vi "Framework Host Sobot.vi"() -> ()   [LabVIEW 2017]
uses:
  TypeDefinitions/TCP Cluster.ctl
  TypeDefinitions/TCP Commands.ctl
  AT901 API/TypeDefinitions/ES_ReflectorType.ctl
  AT901 API/Structures/Struct SystemUnits.ctl
  AT901 API/TypeDefinitions/ES_LengthUnit.ctl
  AT901 API/TypeDefinitions/ES_AngleUnit.ctl
  AT901 API/TypeDefinitions/ES_TemperatureUnit.ctl
  AT901 API/TypeDefinitions/ES_PressureUnit.ctl
  AT901 API/TypeDefinitions/ES_HumidityUnit.ctl
  AT901 API/Structures/Struct EnvironmentData.ctl
  AT901 API/TypeDefinitions/ES_MeasMode.ctl
  AT901 API/TypeDefinitions/ES_CoordinateSystemType.ctl
  AT901 API/Structures/Struct ContinuousTimeModeData.ctl
  AT901 API/TypeDefinitions/ES_RegionType.ctl
  TypeDefinitions/Events.ctl
  <vilib>/Utility/inputDevices.llb/closeJoystick.vi
panel:
  in  "ContinuousTimeModeData":T1={"TimeSeparation"=100, "NumberOfPoints"=0, "UseRegion"=FALSE, "ES_RegionType"=enum."ES_RT_Sphere"}
  in  "Tab Control":enum32{"Allgemein", "Lasertracker"}(tab)
  in  "Button 1":bool
  in  "Button 2":bool
  in  "Manual Drive":bool
  in  "Device Index":i32
  in  "Stop":bool
  out "Send":T3={"Datatype"=enum."Message", "String"="Send to sobot"}
  out "Receive":T3={"Datatype"=enum."Message", "String"="Send to sobot"}
  in  "LT SingleMeasurement":bool
  in  "LT Initialize":bool
  in  "LT GoBirdBath":bool
  in  "LT GetEnvParams":bool
  out "Environmental Data":T5
  in  "LT_SystemUnits":T6
  in  "ES ReflectorType":T12=enum."CCR - 1,5 in"
  in  "LT PowerLock":bool
  out "LT PowerLock Status":bool
  in  "ES_MeasMode":T13
  in  "ES_CoordinateSystemType":T14
  out "Meas Result":dbl[](array[numeric])
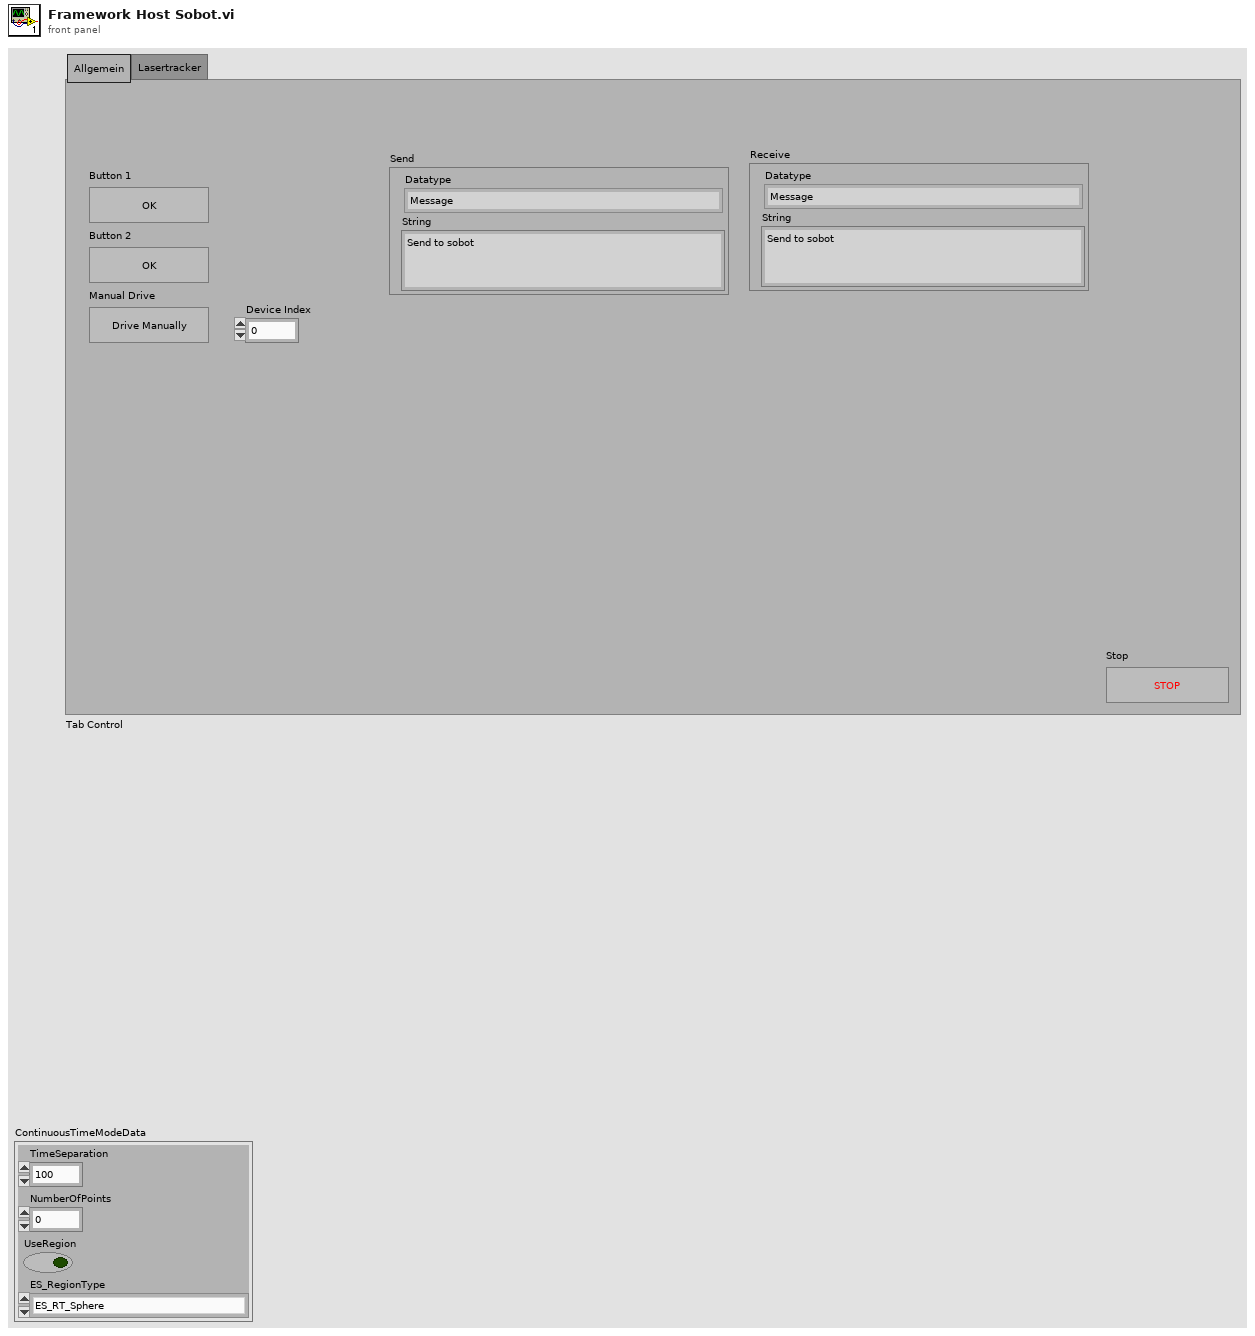
[diagram p1: front panel]
types:
  T1 = typedef "Struct ContinuousTimeModeData.ctl" = cluster{"TimeSeparation":u32, "NumberOfPoints":u32, "UseRegion":bool, "ES_RegionType":T2}
  T2 = typedef "ES_RegionType.ctl" = enum32{"ES_RT_Sphere", "ES_RT_Box"}
  T3 = typedef "TCP Cluster.ctl" = cluster{"Datatype":T4, "String":string}
  T4 = typedef "TCP Commands.ctl" = enum16{"Timeout", "Log", "Message", "ManualDrive", "Stop", "Command"}
  T5 = typedef "Struct EnvironmentData.ctl" = cluster{"Temperature":dbl, "Pressure":dbl, "Humidity":dbl}
  T6 = typedef "Struct SystemUnits.ctl" = cluster{"ES_LengthUnit":T7, "ES_AngleUnit":T8, "ES_TemperatureUnit":T9, "ES_PressureUnit":T10, "ES_HumidityUnit":T11}
  T7 = typedef "ES_LengthUnit.ctl" = enum32{"ES_LU__Meter", "ES_LU_Millimeter", "ES_LU_Micron", "ES_LU_Foot", "ES_LU_Yard", "ES_LU_Inch"}
  T8 = typedef "ES_AngleUnit.ctl" = enum32{"ES_AU_Radian", "ES_AU_Degree", "ES_AU_Gon"}
  T9 = typedef "ES_TemperatureUnit.ctl" = enum32{"ES_TU_Celsius", "ES_TU_Fahrenheit"}
  T10 = typedef "ES_PressureUnit.ctl" = enum32{"ES_PU_Mbar", "ES_PU_HPascal", "ES_PU_KPascal", "ES_PU_MmHg", "ES_PU_Psi", "ES_PU_InH2O", "ES_PU_InHg"}
  T11 = typedef "ES_HumidityUnit.ctl" = enum32{"ES_HU_RH"}
  T12 = typedef "ES_ReflectorType.ctl" = enum32{"none1", "none2", "CCR - 1,5 in", "none4", "none5", "TBR - 0,5 in", "none7", "CCR - 75mm", "none8", "RRR - 1,5 in"}
  T13 = typedef "ES_MeasMode.ctl" = enum32{"ES_MM_Stationary", "ES_MM_ContinuousTime", "ES_MM_ContinuousDistance", "ES_MM_Grid", "ES_MM_SphrereCenter", "ES_MM_CircleCenter", "ES_MM_6DStationary", "ES_MM_6DContinuousTime", "ES_MM_6DContinuousDistance", "ES_MM_6DGrid", "ES_MM_6DSphrereCenter", "ES_MM6DCircleCenter"}
  T14 = typedef "ES_CoordinateSystemType.ctl" = enum32{"ES_CS_RHR", "ES_CS_LHRX", "ES_CS_LHRY", "ES_CS_LHRZ", "ES_CS_CCW", "ES_CS_CCC", "ES_CS_SCW", "ES_CS_SCC"}
  T15 = typedef "Events.ctl" = enum16{"Timeout", "Stop", "Button 1", "Button 2", "StartManualDrive", "ManualDrive", "StopManualDrive", "LT_Initialize", "LT GoBirdBath", "LT_SetReflectorType", "LT_SystemUnits", "LT GetEnvParams", "LT PowerLock", "LT SetMeasMode", "LT SetCoordinateSystemType", "LT SingleMeasurement", "LT SetContinuousTimeModeData"}
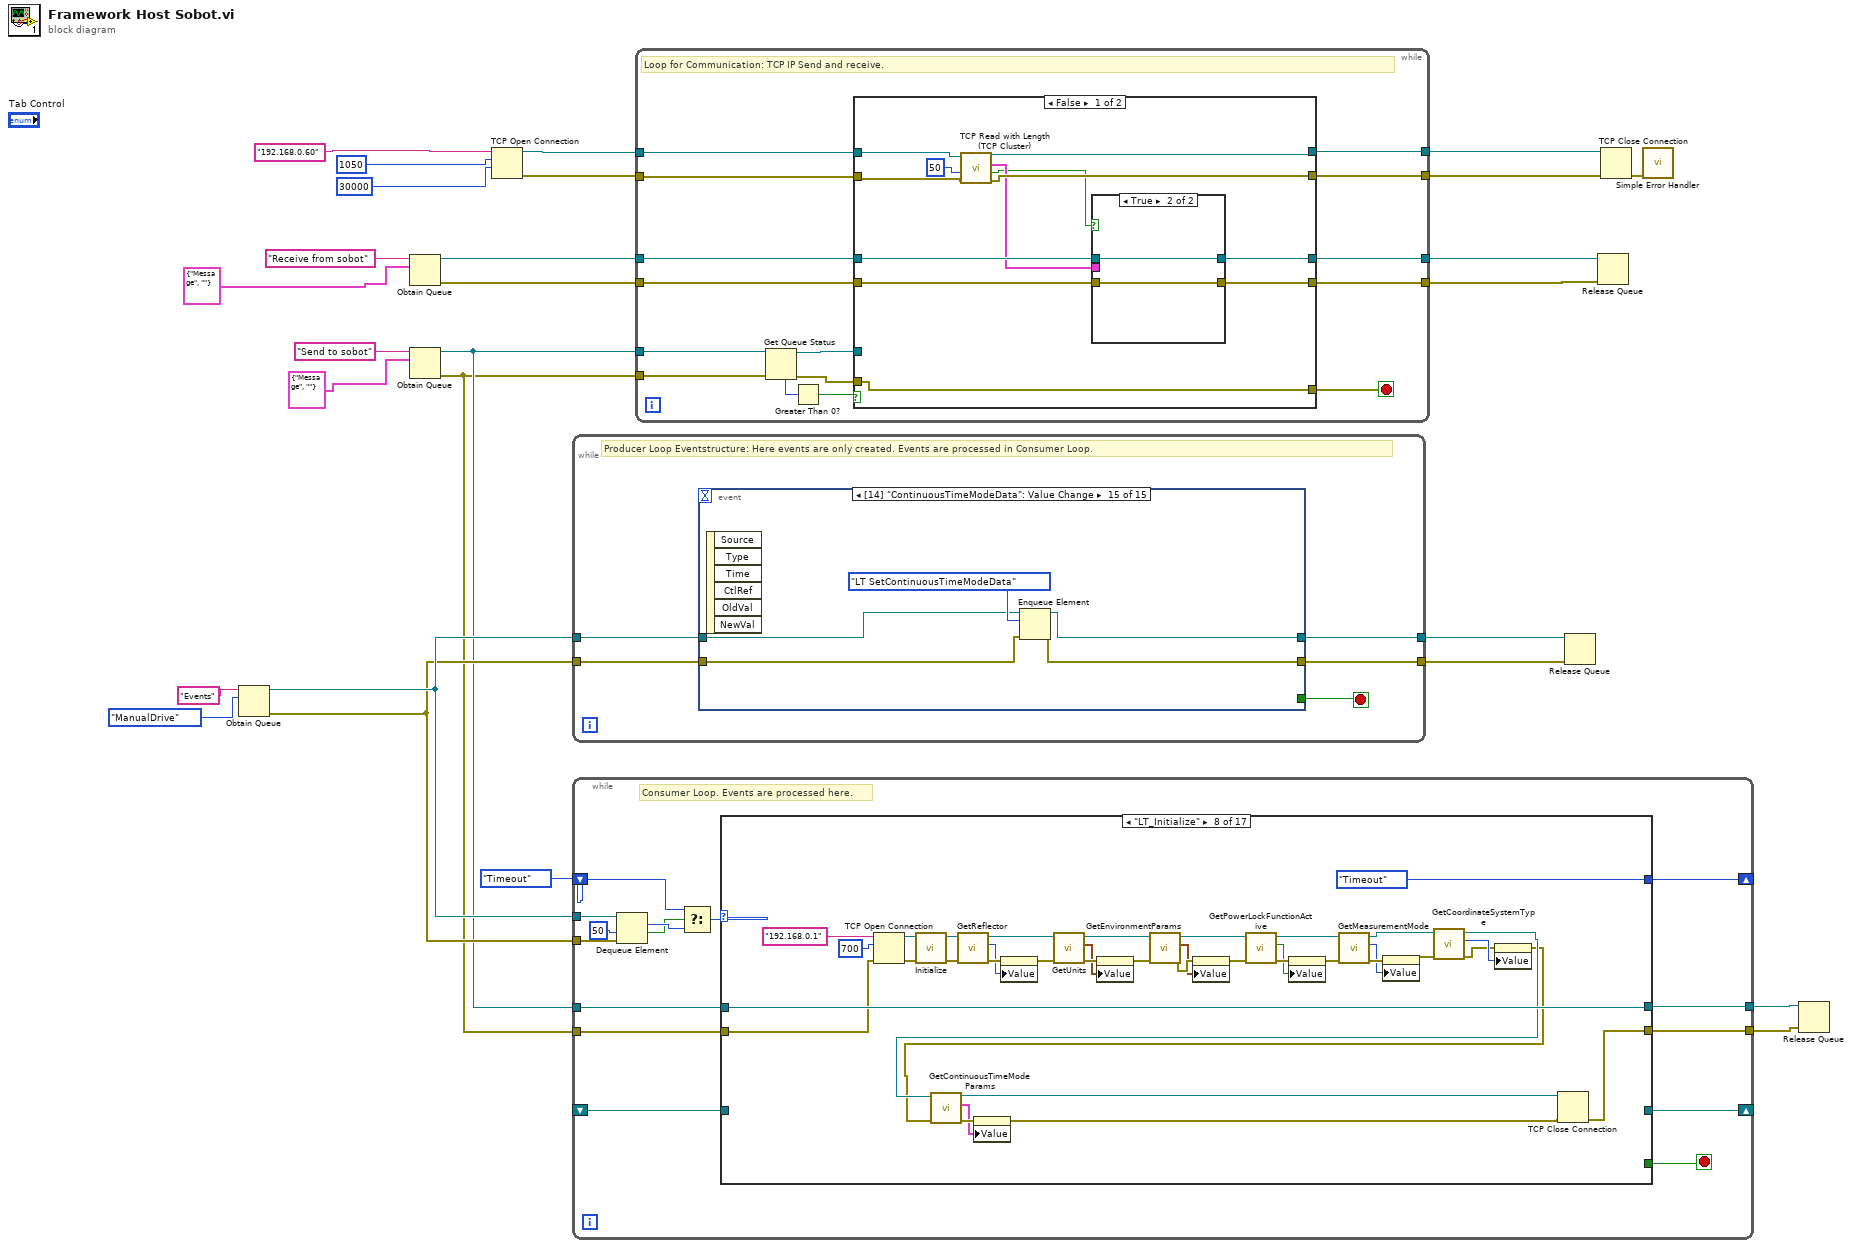
[diagram p0: block diagram]
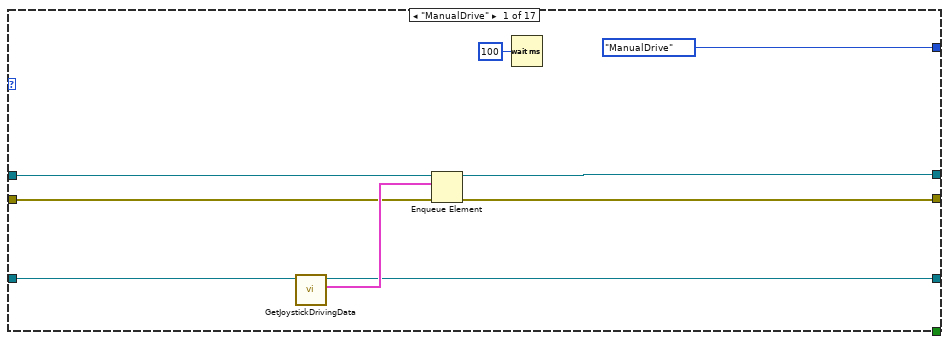
[diagram p2: hidden frame]
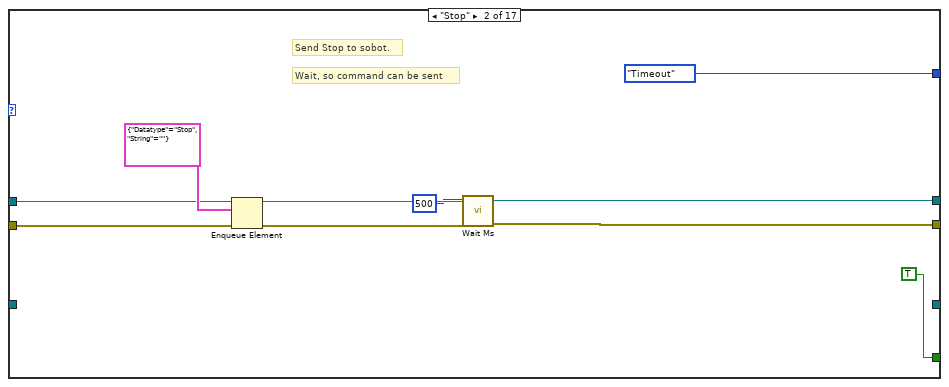
[diagram p3: hidden frame]
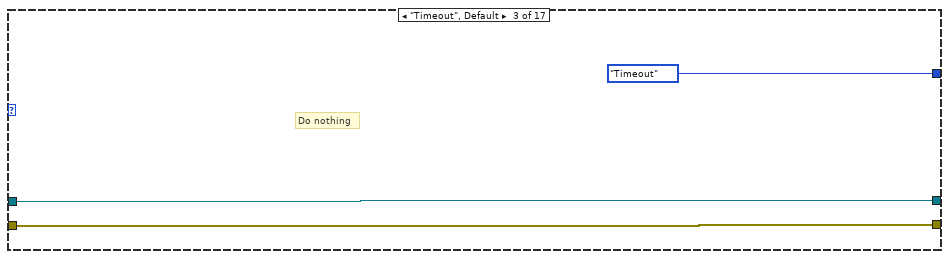
[diagram p4: hidden frame]
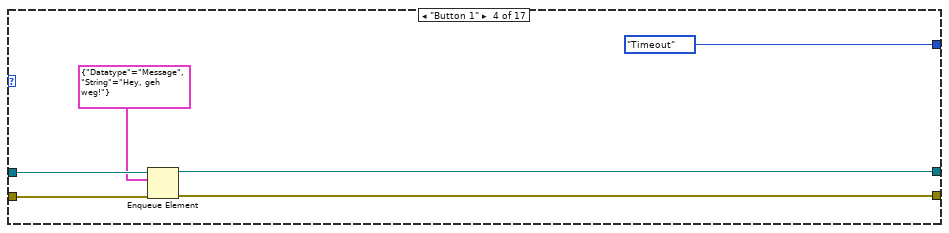
[diagram p5: hidden frame]
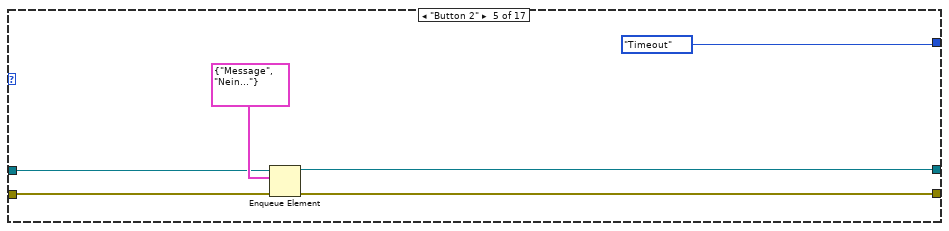
[diagram p6: hidden frame]
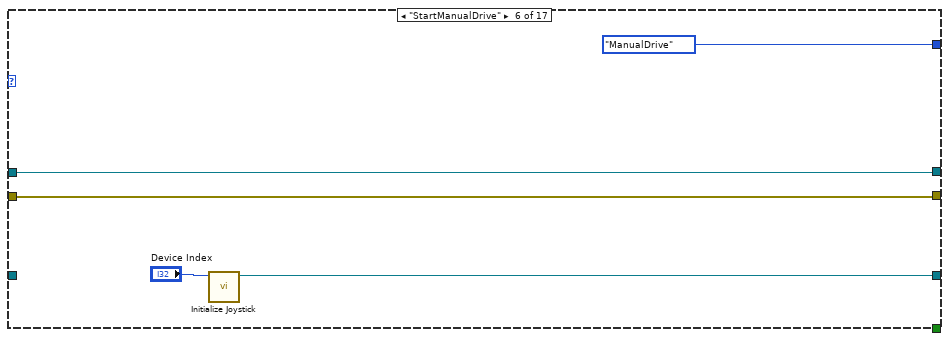
[diagram p7: hidden frame]
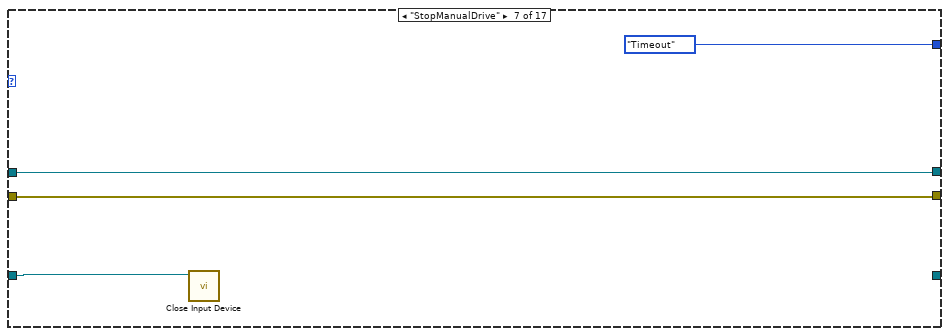
[diagram p8: hidden frame]
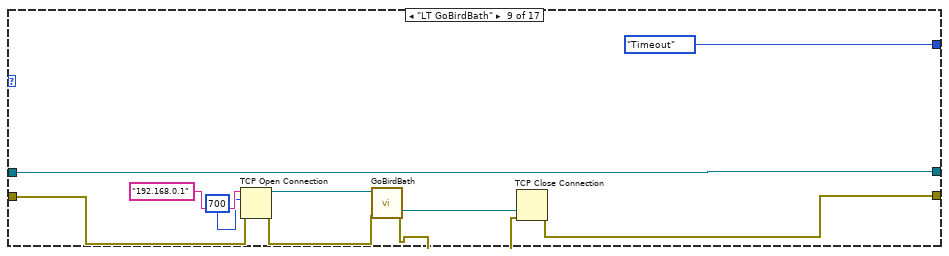
[diagram p9: hidden frame]
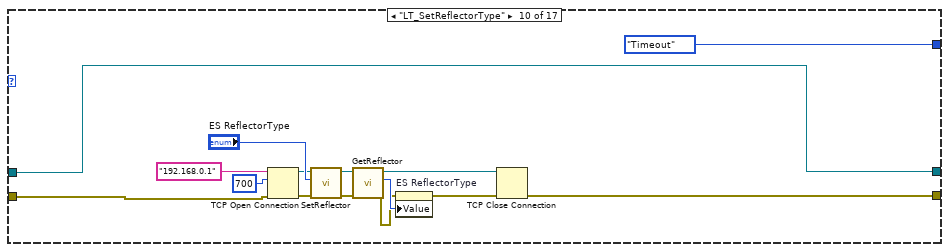
[diagram p10: hidden frame]
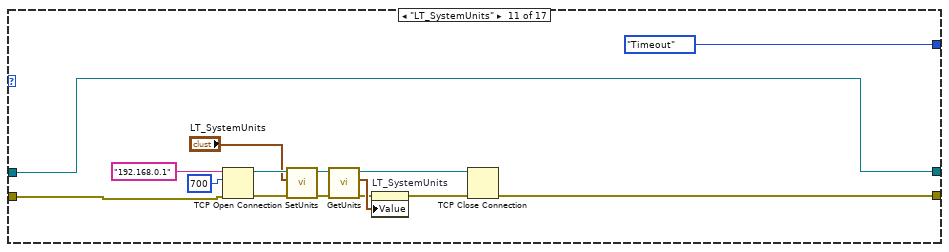
[diagram p11: hidden frame]
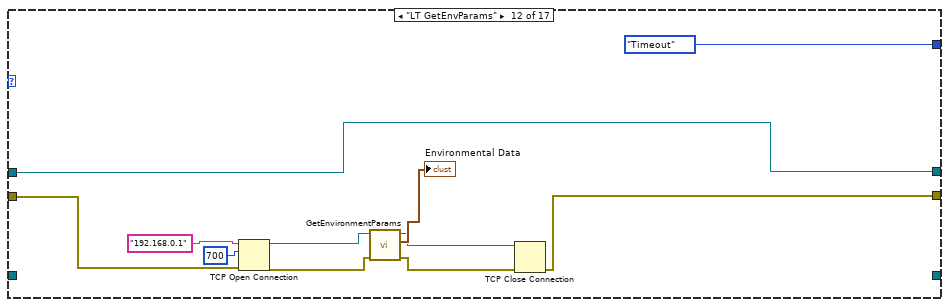
[diagram p12: hidden frame]
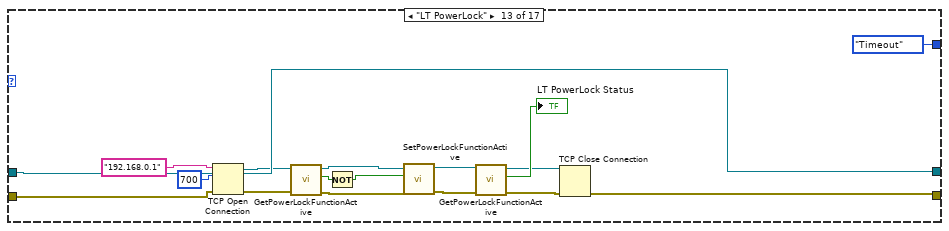
[diagram p13: hidden frame]
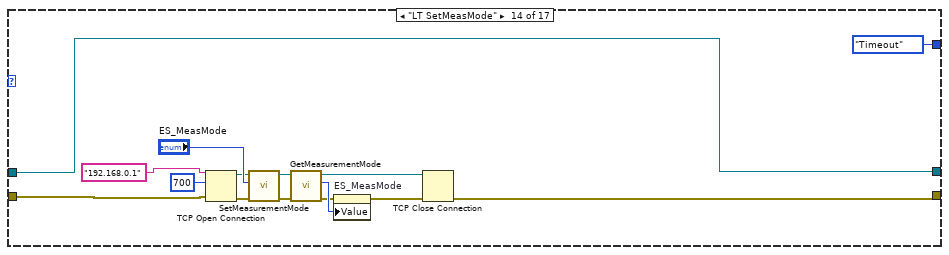
[diagram p14: hidden frame]
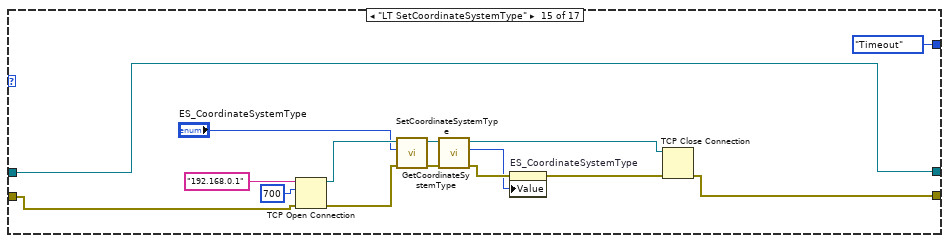
[diagram p15: hidden frame]
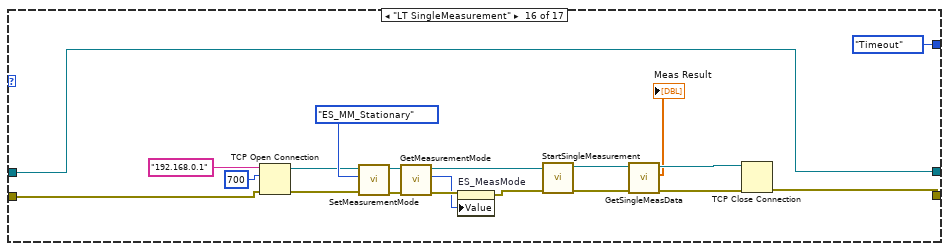
[diagram p16: hidden frame]
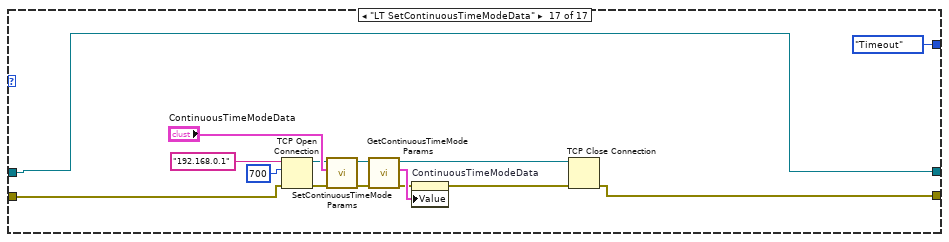
[diagram p17: hidden frame]
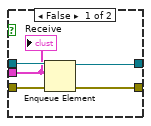
[diagram p18: hidden frame]
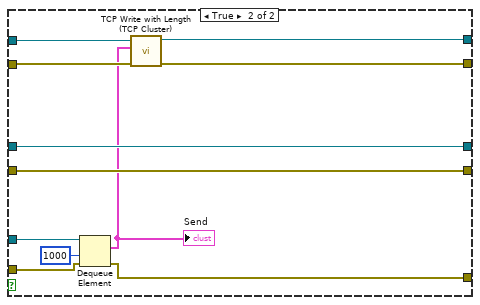
[diagram p19: hidden frame]
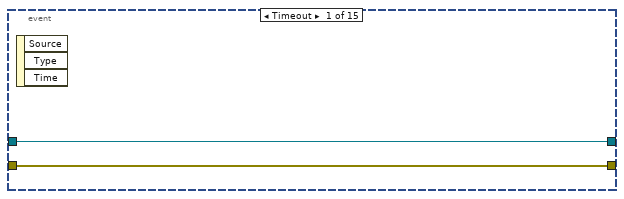
[diagram p20: hidden frame]
diagram:
  n1 = Obtain Queue(name (unnamed)="Events", element data type=Events."ManualDrive" ("Events")) -> (queue out=w7:refnum<queue>, error out=w6:errorcluster)  [unwired: 3 in, 1 out]
  n2 = Obtain Queue(name (unnamed)="Receive from sobot", element data type=T3 {"Datatype"=enum."Message", "String"=""}) -> (queue out=w22:refnum<queue>, error out=w21:errorcluster)  [unwired: 3 in, 1 out]
  n3 = Obtain Queue(name (unnamed)="Send to sobot", element data type=T3 {"Datatype"=enum."Message", "String"=""}) -> (queue out=w4:refnum<queue>, error out=w1:errorcluster)  [unwired: 3 in, 1 out]
  n4 = TCP Open Connection(address="192.168.0.60", remote port or service name=u16 1050, timeout ms (60000)=30000) -> (connection ID=w16:refnum<k5>, error out=w15:errorcluster)  [unwired: 2 in]
  n5 = while {
    tunnel: w7 -> [w31]
    tunnel: w6 -> [w30]
    tunnel: [w29] -> w9
    tunnel: [w28] -> w8
    stop <- w32 stop-if-true
    # "Producer Loop Eventstructure: Here events are only created. Events are processed in Consumer Loop."
    n6 = event shown="[14] \"ContinuousTimeModeData\": Value Change" {
      selector: _ -> [_ _ _ _ _ _ _ _ _ _ _ _ _ _ _]
      dyn-events: _ -> [_ _ _ _ _ _ _ _ _ _ _ _ _ _ _]
      timeout: _ -> [_ _ _ _ _ _ _ _ _ _ _ _ _ _ _]
      tunnel: [_ TRUE _ _ _ _ _ _ _ _ _ _ _ _ _] -> w32
      tunnel: w31 -> [w34 w43 w52 w55 w62 w67 w72 w77 w82 w87 w92 w97 w102 w106 w111]
      tunnel: w30 -> [w33 w41 w51 w56 w61 w66 w71 w76 w79 w86 w91 w96 w101 w105 w108]
      tunnel: [w34 w35 w50 w54 w60 w65 w70 w75 w81 w85 w89 w94 w99 w103 w110] -> w29
      tunnel: [w33 w36 w49 w53 w59 w64 w69 w74 w80 w84 w90 w93 w98 w104 w109] -> w28
      event Timeout {
        n7 = event-data() -> ()  [unwired: 1 in, 3 out]
      }
      event "Stop": Value Change {
        n8 = event-data() -> ()  [unwired: 1 in, 1 out]
        n9 = Enqueue Element(queue=w43, element=Events."Stop" ("Events"), error in (no error)=w41) -> (queue out=w35:refnum<queue>, error out=w39:errorcluster)  [unwired: 1 in, 1 out]
        n10 = call "Wait Ms.vi"("error in (no error)"=w39, "milliseconds to wait"=u32 500) -> ("error out"=w37:errorcluster)  [unwired: 9 in]
        n11 = property on="Stop" class="Bool (strict)"(error in=w37, "Value"=FALSE ("stop")) -> (error out=w36:errorcluster)  [unwired: 1 in, 1 out]
      }
      event "Manual Drive": Value Change {
        n12 = event-data() -> ("OldVal"=w48:bool)  [unwired: 1 in]
        n13 = Select(t=Events."StopManualDrive" ("Events"), s=w48, f=Events."StartManualDrive" ("Events")) -> (s? t:f=w46:T15)
        n14 = Enqueue Element(queue=w52, element=w46, error in (no error)=w51) -> (queue out=w50:refnum<queue>, error out=w49:errorcluster)  [unwired: 1 in, 1 out]
      }
      event "Button 1": Value Change {
        # "Send Example Message"
        n15 = event-data() -> ()  [unwired: 1 in, 1 out]
        n16 = Enqueue Element(queue=w55, element=Events."Button 1" ("Events"), error in (no error)=w56) -> (queue out=w54:refnum<queue>, error out=w53:errorcluster)  [unwired: 1 in, 1 out]
      }
      event "Button 2": Value Change {
        n17 = event-data() -> ()  [unwired: 1 in, 1 out]
        n18 = Enqueue Element(queue=w62, element=Events."Button 2" ("Events"), error in (no error)=w61) -> (queue out=w60:refnum<queue>, error out=w59:errorcluster)  [unwired: 1 in, 1 out]
      }
      event "LT Initialize": Value Change {
        n19 = event-data() -> ()  [unwired: 1 in, 1 out]
        n20 = Enqueue Element(queue=w67, element=Events."LT_Initialize", error in (no error)=w66) -> (queue out=w65:refnum<queue>, error out=w64:errorcluster)  [unwired: 1 in, 1 out]
      }
      event "LT GoBirdBath": Value Change {
        n21 = event-data() -> ()  [unwired: 1 in, 2 out]
        n22 = Enqueue Element(queue=w72, element=Events."LT GoBirdBath" ("Events"), error in (no error)=w71) -> (queue out=w70:refnum<queue>, error out=w69:errorcluster)  [unwired: 1 in, 1 out]
      }
      event Value Change {
        n23 = event-data() -> ()  [unwired: 1 in, 6 out]
        n24 = Enqueue Element(queue=w77, element=Events."LT_SetReflectorType" ("Events"), error in (no error)=w76) -> (queue out=w75:refnum<queue>, error out=w74:errorcluster)  [unwired: 1 in, 1 out]
      }
      event Value Change {
        n25 = event-data() -> ()  [unwired: 1 in, 6 out]
        n26 = Enqueue Element(queue=w82, element=Events."LT_SystemUnits" ("Events"), error in (no error)=w79) -> (queue out=w81:refnum<queue>, error out=w80:errorcluster)  [unwired: 1 in, 1 out]
      }
      event "LT GetEnvParams": Value Change {
        n27 = event-data() -> ()  [unwired: 1 in, 1 out]
        n28 = Enqueue Element(queue=w87, element=Events."LT GetEnvParams" ("Events"), error in (no error)=w86) -> (queue out=w85:refnum<queue>, error out=w84:errorcluster)  [unwired: 1 in, 1 out]
      }
      event "LT PowerLock": Value Change {
        n29 = event-data() -> ()  [unwired: 1 in, 2 out]
        n30 = Enqueue Element(queue=w92, element=Events."LT PowerLock" ("Events"), error in (no error)=w91) -> (queue out=w89:refnum<queue>, error out=w90:errorcluster)  [unwired: 1 in, 1 out]
      }
      event "LT SingleMeasurement": Value Change {
        n31 = event-data() -> ()  [unwired: 1 in, 1 out]
        n32 = Enqueue Element(queue=w97, element=Events."LT SingleMeasurement", error in (no error)=w96) -> (queue out=w94:refnum<queue>, error out=w93:errorcluster)  [unwired: 1 in, 1 out]
      }
      event Value Change {
        n33 = event-data() -> ()  [unwired: 1 in, 1 out]
        n34 = Enqueue Element(queue=w102, element=Events."LT SetMeasMode", error in (no error)=w101) -> (queue out=w99:refnum<queue>, error out=w98:errorcluster)  [unwired: 1 in, 1 out]
      }
      event Value Change {
        n35 = event-data() -> ()  [unwired: 1 in, 6 out]
        n36 = Enqueue Element(queue=w106, element=Events."LT SetCoordinateSystemType", error in (no error)=w105) -> (queue out=w103:refnum<queue>, error out=w104:errorcluster)  [unwired: 1 in, 1 out]
      }
      event Value Change {
        n37 = event-data() -> ()  [unwired: 1 in, 6 out]
        n38 = Enqueue Element(queue=w111, element=Events."LT SetContinuousTimeModeData", error in (no error)=w108) -> (queue out=w110:refnum<queue>, error out=w109:errorcluster)  [unwired: 1 in, 1 out]
      }
    }
  }
  n39 = while {
    tunnel: w7 -> [w127]
    tunnel: w6 -> [w126]
    shift-right: [w123] -> _
    shift-left: Events."Timeout" ("Events") -> [w122]
    tunnel: w4 -> [w118]
    tunnel: [w117] -> w3
    tunnel: [w116] -> w2
    tunnel: w1 -> [w115]
    shift-right: [w114] -> _
    shift-left: _ -> [w113]
    stop <- w124 stop-if-true
    # "Consumer Loop. Events are processed here."
    n40 = Dequeue Element(queue=w127, timeout in ms (-1)=50, error in (no error)=w126) -> (element=w121:T15, timed out?=w119:bool)  [unwired: 2 out]
    n41 = Select(t=w122, s=w119, f=w121) -> (s? t:f=w120:T15)
    n42 = case shown="\"LT_Initialize\"" w120 {
      tunnel: [_ TRUE _ _ _ _ _ _ _ _ _ _ _ _ _ _ _] -> w124
      tunnel: [Events."ManualDrive" ("Events") Events."Timeout" ("Events") Events."Timeout" ("Events") Events."Timeout" ("Events") Events."Timeout" ("Events") Events."ManualDrive" ("Events") Events."Timeout" ("Events") Events."Timeout" ("Events") Events."Timeout" ("Events") Events."Timeout" ("Events") Events."Timeout" ("Events") Events."Timeout" ("Events") Events."Timeout" ("Events") Events."Timeout" ("Events") Events."Timeout" ("Events") Events."Timeout" ("Events") Events."Timeout" ("Events")] -> w123
      tunnel: w118 -> [w134 w142 w147 w154 w159 w165 w168 w207 w210 w218 w234 w249 w273 w284 w305 w321 w328]
      tunnel: [w133 w141 w147 w151 w157 w165 w168 w207 w210 w218 w234 w249 w273 w284 w305 w321 w328] -> w117
      tunnel: [w128 w138 w146 w150 w156 w164 w167 w200 w211 w223 w235 w250 w272 w285 w302 w322 w326] -> w116
      tunnel: w115 -> [w129 w137 w146 w153 w158 w164 w167 w201 w212 w224 w236 w251 w271 w286 w293 w323 w329]
      tunnel: [w132 _ _ _ _ w162 _ _ _ _ _ _ _ _ _ _ _] -> w114
      tunnel: w113 -> [w131 _ _ _ _ _ w169 _ _ _ _ _ _ _ _ _ _]
      frame "ManualDrive" {
        n43 = call "GetJoystickDrivingData.vi"("Refnum in"=w131) -> ("DriveData"=w136:T3, "Refnum out"=w132:refnum<k1>)  [unwired: 6 in, 3 out]
        n44 = Enqueue Element(queue=w134, element=w136, error in (no error)=w129) -> (queue out=w133:refnum<queue>, error out=w128:errorcluster)  [unwired: 1 in, 1 out]
        n45 = Wait (ms)(milliseconds to wait=u32 100) -> ()  [unwired: 1 out]
      }
      frame "Stop" {
        # "Wait, so command can be sent"
        # "Send Stop to sobot."
        n46 = Enqueue Element(queue=w142, element=T3 {"Datatype"=enum."Stop", "String"=""}, error in (no error)=w137) -> (queue out=w141:refnum<queue>, error out=w139:errorcluster)  [unwired: 1 in, 1 out]
        n47 = call "Wait Ms.vi"("error in (no error)"=w139, "milliseconds to wait"=u32 500) -> ("error out"=w138:errorcluster)  [unwired: 9 in]
      }
      frame "Timeout", Default {
        # "Do nothing"
      }
      frame "Button 1" {
        n48 = Enqueue Element(queue=w154, element=T3 {"Datatype"=enum."Message", "String"="Hey, geh weg!"}, error in (no error)=w153) -> (queue out=w151:refnum<queue>, error out=w150:errorcluster)  [unwired: 1 in, 1 out]
      }
      frame "Button 2" {
        n49 = Enqueue Element(queue=w159, element=T3 {"Datatype"=enum."Message", "String"="Nein..."}, error in (no error)=w158) -> (queue out=w157:refnum<queue>, error out=w156:errorcluster)  [unwired: 1 in, 1 out]
      }
      frame "StartManualDrive" {
        n50 = call <vilib>:"Initialize Joystick.vi"("device index"="Device Index") -> ("device ID"=w162:refnum<k1>)  [unwired: 9 in, 1 out]
      }
      frame "StopManualDrive" {
        n51 = call-poly <vilib>:"Close Input Device.vi"("device ID"=w169) -> ()  [unwired: 9 in, 1 out]
      }
      frame "LT_Initialize" {
        n52 = TCP Open Connection(address="192.168.0.1", remote port or service name=u16 700, error in (no error)=w201) -> (connection ID=w203:refnum<k5>, error out=w202:errorcluster)  [unwired: 2 in]
        n53 = call "Initialize.vi"("error in (no error)"=w202, "TCP Network Connection in"=w203) -> ("error out"=w198:errorcluster, "TCP Network Connection out"=w199:refnum<k5>)  [unwired: 6 in, 2 out]
        n54 = call "GetReflector.vi"("error in (no error)"=w198, "TCP Network Connection in"=w199) -> ("error out"=w197:errorcluster, "ES ReflectorType"=w196:T12, "TCP Network Connection out"=w184:refnum<k5>)  [unwired: 5 in, 2 out]
        n55 = property on="ES ReflectorType" class="Enum (strict)"(error in=w197, "Value"=w196) -> (error out=w185:errorcluster)  [unwired: 1 in, 1 out]
        n56 = call "GetUnits.vi"("error in (no error)"=w185, "TCP Network Connection in"=w184) -> ("error out"=w187:errorcluster, "SystemUnits"=w186:T6, "TCP Network Connection out"=w195:refnum<k5>)  [unwired: 5 in, 2 out]
        n57 = property on="LT_SystemUnits" class="Clust (strict)"(error in=w187, "Value"=w186) -> (error out=w190:errorcluster)  [unwired: 1 in, 1 out]
        n58 = call "GetEnvironmentParams.vi"("error in (no error)"=w190, "TCP Network Connection in"=w195) -> ("error out"=w189:errorcluster, "Environmental Data"=w188:T5, "TCP Network Connection out"=w194:refnum<k5>)  [unwired: 5 in, 2 out]
        n59 = property on="Environmental Data" class="Clust (strict)"(error in=w189, "Value"=w188) -> (error out=w193:errorcluster)  [unwired: 1 in, 1 out]
        n60 = call "GetPowerLockFunctionActive.vi"("error in (no error)"=w193, "TCP Network Connection in"=w194) -> ("error out"=w192:errorcluster, "ES_BOOL"=w191:bool, "TCP Network Connection out"=w181:refnum<k5>)  [unwired: 5 in, 2 out]
        n61 = property on="LT PowerLock Status" class="Bool (strict)"(error in=w192, "Value"=w191) -> (error out=w180:errorcluster)  [unwired: 1 in, 1 out]
        n62 = call "GetMeasurementMode.vi"("error in (no error)"=w180, "TCP Network Connection in"=w181) -> ("error out"=w183:errorcluster, "ES_MeasMode"=w182:T13, "TCP Network Connection out"=w177:refnum<k5>)  [unwired: 5 in, 2 out]
        n63 = property on="ES_MeasMode" class="Enum (strict)"(error in=w183, "Value"=w182) -> (error out=w176:errorcluster)  [unwired: 1 in, 1 out]
        n64 = call "GetCoordinateSystemType.vi"("error in (no error)"=w176, "TCP Network Connection in"=w177) -> ("error out"=w178:errorcluster, "ES_CoordinateSystemType"=w179:T14, "TCP Network Connection out"=w173:refnum<k5>)  [unwired: 5 in, 2 out]
        n65 = property on="ES_CoordinateSystemType" class="Enum (strict)"(error in=w178, "Value"=w179) -> (error out=w172:errorcluster)  [unwired: 1 in, 1 out]
        n66 = call "GetContinuousTimeModeParams.vi"("error in (no error)"=w172, "TCP Network Connection in"=w173) -> ("error out"=w175:errorcluster, "ContinuousTimeModeData"=w174:T1, "TCP Network Connection out"=w170:refnum<k5>)  [unwired: 5 in, 2 out]
        n67 = property on="ContinuousTimeModeData" class="Clust (strict)"(error in=w175, "Value"=w174) -> (error out=w171:errorcluster)  [unwired: 1 in, 1 out]
        n68 = TCP Close Connection(connection ID=w170, error in (no error)=w171) -> (error out=w200:errorcluster)  [unwired: 1 in, 1 out]
      }
      frame "LT GoBirdBath" {
        n69 = TCP Open Connection(address="192.168.0.1", remote port or service name=u16 700, error in (no error)=w212) -> (connection ID=w215:refnum<k5>, error out=w214:errorcluster)  [unwired: 2 in]
        n70 = call "GoBirdBath.vi"("error in (no error)"=w214, "TCP Network Connection in"=w215) -> ("error out"=w208:errorcluster, "TCP Network Connection out"=w213:refnum<k5>)  [unwired: 6 in, 2 out]
        n71 = TCP Close Connection(connection ID=w213, error in (no error)=w208) -> (error out=w211:errorcluster)  [unwired: 1 in, 1 out]
      }
      frame "LT_SetReflectorType" {
        n72 = TCP Open Connection(address="192.168.0.1", remote port or service name=u16 700, error in (no error)=w224) -> (connection ID=w227:refnum<k5>, error out=w231:errorcluster)  [unwired: 2 in]
        n73 = call "SetReflector.vi"("error in (no error)"=w231, "ES ReflectorType"="ES ReflectorType", "TCP Network Connection in"=w227) -> ("error out"=w230:errorcluster, "TCP Network Connection out"=w229:refnum<k5>)  [unwired: 5 in, 2 out]
        n74 = call "GetReflector.vi"("error in (no error)"=w230, "TCP Network Connection in"=w229) -> ("error out"=w220:errorcluster, "ES ReflectorType"=w221:T12, "TCP Network Connection out"=w228:refnum<k5>)  [unwired: 5 in, 2 out]
        n75 = property on="ES ReflectorType" class="Enum (strict)"(error in=w220, "Value"=w221) -> (error out=w219:errorcluster)  [unwired: 1 in, 1 out]
        n76 = TCP Close Connection(connection ID=w228, error in (no error)=w219) -> (error out=w223:errorcluster)  [unwired: 1 in, 1 out]
      }
      frame "LT_SystemUnits" {
        n77 = TCP Open Connection(address="192.168.0.1", remote port or service name=u16 700, error in (no error)=w236) -> (connection ID=w242:refnum<k5>, error out=w246:errorcluster)  [unwired: 2 in]
        n78 = call "SetUnits.vi"("error in (no error)"=w246, "SystemUnits"="LT_SystemUnits", "TCP Network Connection in"=w242) -> ("error out"=w245:errorcluster, "TCP Network Connection out"=w243:refnum<k5>)  [unwired: 5 in, 2 out]
        n79 = call "GetUnits.vi"("error in (no error)"=w245, "TCP Network Connection in"=w243) -> ("error out"=w238:errorcluster, "SystemUnits"=w247:T6, "TCP Network Connection out"=w244:refnum<k5>)  [unwired: 5 in, 2 out]
        n80 = property on="LT_SystemUnits" class="Clust (strict)"(error in=w238, "Value"=w247) -> (error out=w237:errorcluster)  [unwired: 1 in, 1 out]
        n81 = TCP Close Connection(connection ID=w244, error in (no error)=w237) -> (error out=w235:errorcluster)  [unwired: 1 in, 1 out]
      }
      frame "LT GetEnvParams" {
        n82 = TCP Open Connection(address="192.168.0.1", remote port or service name=u16 700, error in (no error)=w251) -> (connection ID=w254:refnum<k5>, error out=w257:errorcluster)  [unwired: 2 in]
        n83 = call "GetEnvironmentParams.vi"("error in (no error)"=w257, "TCP Network Connection in"=w254) -> ("error out"=w256:errorcluster, "Environmental Data"=→"Environmental Data":T5, "TCP Network Connection out"=w255:refnum<k5>)  [unwired: 5 in, 2 out]
        n84 = TCP Close Connection(connection ID=w255, error in (no error)=w256) -> (error out=w250:errorcluster)  [unwired: 1 in, 1 out]
      }
      frame "LT PowerLock" {
        n85 = TCP Open Connection(address="192.168.0.1", remote port or service name=u16 700, error in (no error)=w271) -> (connection ID=w268:refnum<k5>, error out=w264:errorcluster)  [unwired: 2 in]
        n86 = call "GetPowerLockFunctionActive.vi"("error in (no error)"=w264, "TCP Network Connection in"=w268) -> ("error out"=w265:errorcluster, "ES_BOOL"=w267:bool, "TCP Network Connection out"=w269:refnum<k5>)  [unwired: 5 in, 2 out]
        n87 = Not(x=w267) -> (.not. x?=w266:bool)
        n88 = call "SetPowerLockFunctionActive.vi"("error in (no error)"=w265, "ES_BOOL"=w266, "TCP Network Connection in"=w269) -> ("error out"=w262:errorcluster, "TCP Network Connection out"=w263:refnum<k5>)  [unwired: 5 in, 2 out]
        n89 = call "GetPowerLockFunctionActive.vi"("error in (no error)"=w262, "TCP Network Connection in"=w263) -> ("error out"=w259:errorcluster, "ES_BOOL"=→"LT PowerLock Status":bool, "TCP Network Connection out"=w260:refnum<k5>)  [unwired: 5 in, 2 out]
        n90 = TCP Close Connection(connection ID=w260, error in (no error)=w259) -> (error out=w272:errorcluster)  [unwired: 1 in, 1 out]
      }
      frame "LT SetMeasMode" {
        n91 = TCP Open Connection(address="192.168.0.1", remote port or service name=u16 700, error in (no error)=w286) -> (connection ID=w278:refnum<k5>, error out=w288:errorcluster)  [unwired: 2 in]
        n92 = call "SetMeasurementMode.vi"("error in (no error)"=w288, "ES_MeasMode"="ES_MeasMode", "TCP Network Connection in"=w278) -> ("error out"=w289:errorcluster, "TCP Network Connection out"=w280:refnum<k5>)  [unwired: 5 in, 2 out]
        n93 = call "GetMeasurementMode.vi"("error in (no error)"=w289, "TCP Network Connection in"=w280) -> ("error out"=w282:errorcluster, "ES_MeasMode"=w283:T13, "TCP Network Connection out"=w279:refnum<k5>)  [unwired: 5 in, 2 out]
        n94 = property on="ES_MeasMode" class="Enum (strict)"(error in=w282, "Value"=w283) -> (error out=w281:errorcluster)  [unwired: 1 in, 1 out]
        n95 = TCP Close Connection(connection ID=w279, error in (no error)=w281) -> (error out=w285:errorcluster)  [unwired: 1 in, 1 out]
      }
      frame "LT SetCoordinateSystemType" {
        n96 = TCP Open Connection(address="192.168.0.1", remote port or service name=u16 700, error in (no error)=w293) -> (connection ID=w298:refnum<k5>, error out=w297:errorcluster)  [unwired: 2 in]
        n97 = call "SetCoordinateSystemType.vi"("error in (no error)"=w297, "ES_CoordinateSystemType"="ES_CoordinateSystemType", "TCP Network Connection in"=w298) -> ("error out"=w301:errorcluster, "TCP Network Connection out"=w291:refnum<k5>)  [unwired: 5 in, 2 out]
        n98 = call "GetCoordinateSystemType.vi"("error in (no error)"=w301, "TCP Network Connection in"=w291) -> ("error out"=w296:errorcluster, "ES_CoordinateSystemType"=w295:T14, "TCP Network Connection out"=w292:refnum<k5>)  [unwired: 5 in, 2 out]
        n99 = property on="ES_CoordinateSystemType" class="Enum (strict)"(error in=w296, "Value"=w295) -> (error out=w303:errorcluster)  [unwired: 1 in, 1 out]
        n100 = TCP Close Connection(connection ID=w292, error in (no error)=w303) -> (error out=w302:errorcluster)  [unwired: 1 in, 1 out]
      }
      frame "LT SingleMeasurement" {
        n101 = TCP Open Connection(address="192.168.0.1", remote port or service name=u16 700, error in (no error)=w323) -> (connection ID=w313:refnum<k5>, error out=w312:errorcluster)  [unwired: 2 in]
        n102 = call "SetMeasurementMode.vi"("error in (no error)"=w312, "ES_MeasMode"=ES_MeasMode."ES_MM_Stationary", "TCP Network Connection in"=w313) -> ("error out"=w320:errorcluster, "TCP Network Connection out"=w319:refnum<k5>)  [unwired: 5 in, 2 out]
        n103 = call "GetMeasurementMode.vi"("error in (no error)"=w320, "TCP Network Connection in"=w319) -> ("error out"=w317:errorcluster, "ES_MeasMode"=w315:T13, "TCP Network Connection out"=w314:refnum<k5>)  [unwired: 5 in, 2 out]
        n104 = property on="ES_MeasMode" class="Enum (strict)"(error in=w317, "Value"=w315) -> (error out=w316:errorcluster)  [unwired: 1 in, 1 out]
        n105 = call "StartSingleMeasurement.vi"("error in (no error)"=w316, "TCP Network Connection in"=w314) -> ("error out"=w309:errorcluster, "TCP Network Connection out"=w310:refnum<k5>)  [unwired: 7 in, 1 out]
        n106 = call "GetSingleMeasData.vi"("error in (no error)"=w309, "TCP Network Connection in"=w310) -> ("error out"=w308:errorcluster, "Meas Result"=→"Meas Result":dbl[], "TCP Network Connection out"=w307:refnum<k5>)  [unwired: 6 in, 1 out]
        n107 = TCP Close Connection(connection ID=w307, error in (no error)=w308) -> (error out=w322:errorcluster)  [unwired: 1 in, 1 out]
      }
      frame "LT SetContinuousTimeModeData" {
        n108 = TCP Open Connection(address="192.168.0.1", remote port or service name=u16 700, error in (no error)=w329) -> (connection ID=w332:refnum<k5>, error out=w333:errorcluster)  [unwired: 2 in]
        n109 = call "SetContinuousTimeModeParams.vi"("error in (no error)"=w333, "ContinuousTimeModeData"="ContinuousTimeModeData", "TCP Network Connection in"=w332) -> ("error out"=w335:errorcluster, "TCP Network Connection out"=w334:refnum<k5>)  [unwired: 5 in, 2 out]
        n110 = call "GetContinuousTimeModeParams.vi"("error in (no error)"=w335, "TCP Network Connection in"=w334) -> ("error out"=w338:errorcluster, "ContinuousTimeModeData"=w340:T1, "TCP Network Connection out"=w336:refnum<k5>)  [unwired: 5 in, 2 out]
        n111 = property on="ContinuousTimeModeData" class="Clust (strict)"(error in=w338, "Value"=w340) -> (error out=w339:errorcluster)  [unwired: 1 in, 1 out]
        n112 = TCP Close Connection(connection ID=w336, error in (no error)=w339) -> (error out=w326:errorcluster)  [unwired: 1 in, 1 out]
      }
    }
  }
  n113 = while {
    tunnel: w4 -> [w354]
    tunnel: w1 -> [w352]
    tunnel: w16 -> [w348]
    tunnel: w15 -> [w347]
    tunnel: [w346] -> w25
    tunnel: [w345] -> w24
    tunnel: w22 -> [w344]
    tunnel: w21 -> [w343]
    tunnel: [w342] -> w19
    tunnel: [w341] -> w20
    stop <- w355 stop-if-true
    # "Loop for Communication: TCP IP Send and receive."
    n114 = Get Queue Status(queue=w354, error in (no error)=w352) -> (queue out=w353:refnum<queue>, error out=w351:errorcluster, # elements in queue=w350:i32)  [unwired: 1 in, 5 out]
    n115 = Greater Than 0?(x=w350) -> (x > 0?=w349:bool)
    n116 = case shown="False" w349 {
      tunnel: [w367 w385] -> w355
      tunnel: w353 -> [_ w383]
      tunnel: w351 -> [w367 w382]
      tunnel: w348 -> [w362 w379]
      tunnel: w347 -> [w361 w378]
      tunnel: [w359 w377] -> w345
      tunnel: [w358 w376] -> w346
      tunnel: w344 -> [w366 w381]
      tunnel: w343 -> [w365 w380]
      tunnel: [w364 w381] -> w341
      tunnel: [w363 w380] -> w342
      frame False {
        n117 = call "TCP Read with Length (TCP Cluster).vi"("error in (no error)"=w361, "Timeout"=50, "connection ID"=w362) -> ("error out"=w359:errorcluster, "Timeout?"=w356:bool, "TCP Cluster"=w357:T3, "connection ID out"=w358:refnum<k5>)  [unwired: 5 in]
        n118 = case shown="True" w356 {
          tunnel: w366 -> [w372 w374]
          tunnel: w365 -> [w371 w373]
          tunnel: w357 -> [w370 _]
          tunnel: [w369 w374] -> w364
          tunnel: [w368 w373] -> w363
          frame False {
            n119 = Enqueue Element(queue=w372, element=w370, error in (no error)=w371) -> (queue out=w369:refnum<queue>, error out=w368:errorcluster)  [unwired: 1 in, 1 out]
            "Receive" <- w370
          }
          frame True {
          }
        }
      }
      frame True {
        n120 = Dequeue Element(queue=w383, timeout in ms (-1)=1000, error in (no error)=w382) -> (element=w375:T3, error out=w385:errorcluster)  [unwired: 2 out]
        "Send" <- w375
        n121 = call "TCP Write with Length (TCP Cluster).vi"("error in (no error)"=w378, 10:w375, "connection ID"=w379) -> ("error out"=w377:errorcluster, "connection ID out"=w376:refnum<k5>)  [unwired: 7 in]
      }
    }
  }
  n122 = Release Queue(queue=w9, error in (no error)=w8) -> ()  [unwired: 1 in, 3 out]
  n123 = Release Queue(queue=w20, error in (no error)=w19) -> ()  [unwired: 1 in, 3 out]
  n124 = TCP Close Connection(connection ID=w25, error in (no error)=w24) -> (error out=w26:errorcluster)  [unwired: 1 in, 1 out]
  n125 = call <vilib>:"Simple Error Handler.vi"("error in (no error)"=w26) -> ()  [unwired: 4 in, 5 out]
  n126 = Release Queue(queue=w3, error in (no error)=w2) -> ()  [unwired: 1 in, 3 out]
